vi "종료.vi"(8 "error in":errorcluster) -> (0 "error out":errorcluster)   [LabVIEW 2023]
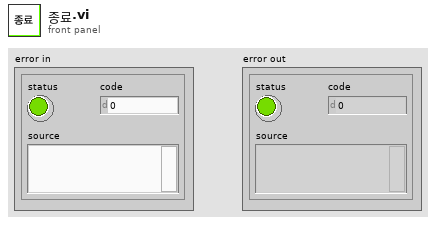
[diagram p1: front panel]
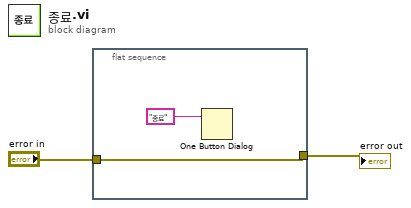
[diagram p0: block diagram]
diagram:
  n1 = flat-sequence {
    tunnel: [w3] -> w1
    tunnel: "error in" -> [w3]
    frame #0 {
      n2 = One Button Dialog(message="종료") -> ()  [unwired: 1 in, 1 out]
    }
  }
  "error out" <- w1
